vi "Binary MLS.vi"(7 "initialize?":bool=TRUE, 9 "seed":i64=-1 format="%.0x", 10 "polynomial order":i32=31 max=512, 11 "samples":i64=128) -> (0 "error code":i32, 3 "mls sequence":u8[](array[numeric]))   [LabVIEW 2020, in "NI_AALBase.lvlib"]
doc: "Generates a maximum length sequence of ones and zeros using a modulo-2 primitive polynomial of order <B>polynomial order</B>."
uses:
  NI_AALBase.lvlib
panel:
  # "Binary MLS"
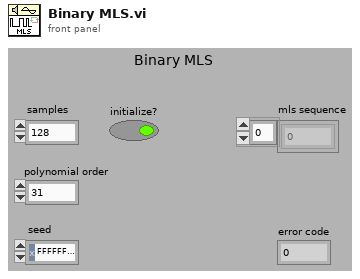
[diagram p1: front panel]
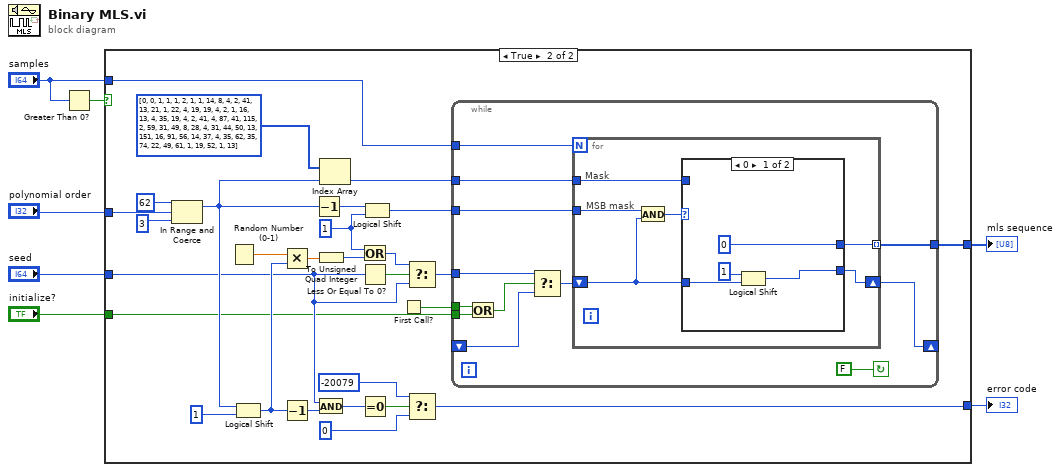
[diagram p0: block diagram]
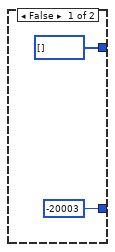
[diagram p2: hidden frame]
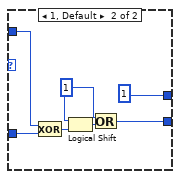
[diagram p3: hidden frame]
diagram:
  n1 = Greater Than 0?(x="samples") -> (x > 0?=w2:bool)
  n2 = case shown="True" w2 {
    tunnel: "polynomial order" -> [_ w35]
    tunnel: "samples" -> [_ w31]
    tunnel: [u8[] [] w28] -> w6
    tunnel: [-20003 ("t") w22] -> w5
    tunnel: "seed" -> [_ w14]
    tunnel: "initialize?" -> [_ w13]
    frame False {
    }
    frame True {
      w16 = u64 1 ("y")
      n3 = In Range and Coerce(upper limit=u16 62, x=w35, lower limit=u16 3) -> (coerced(x)=w25:i32)  [unwired: 1 out]
      n4 = Random Number (0-1)() -> (number: 0 to 1=w18:dbl)
      n5 = Logical Shift(y=w25, x=u64 1 ("y")) -> (x << y=w17:u64)
      n6 = Multiply(x=w18, y=w17) -> (x*y=w20:dbl)
      n7 = Decrement(x=w17) -> (x-1=w26:u64)
      n8 = Decrement(x=w25) -> (x-1=w32:i32)
      n9 = To Unsigned Quad Integer(1:w20) -> (0:w19:u64)
      n10 = And(x=w14, y=w26) -> (x .and. y?=w29:u64)
      n11 = Index Array(array=u64[] [0, 0, 1, 1, 1, 2, 1, 1, 14, 8, 4, 2, 41, 13, 21, 1, 22, 4, 19, 19, 4, 2, 1, 16, 13, 4, 35, 19, 4, 2, 41, 4, 87, 41, 115, 2, 59, 31, 49, 8, 28, 4, 31, 44, 50, 13, 151, 16, 91, 56, 14, 37, 4, 35, 62, 35, 74, 22, 49, 61, 1, 19, 52, 1, 13] ("appended array"), index=w25) -> (element=w34:u64)
      n12 = Or(x=w16, y=w19) -> (x .or. y?=w10:u64)
      n13 = Less Or Equal To 0?(x=w14) -> (x <= 0?=w15:bool)
      n14 = Equal To 0?(x=w29) -> (x = 0?=w24:bool)
      n15 = Logical Shift(y=w32, x=w16) -> (x << y=w33:u64)
      n16 = First Call?() -> (First Call?: T/F=w12:bool)
      n17 = Select(t=w10, s=w15, f=w14) -> (s? t:f=w11:u64)
      n18 = Select(t=-20079, s=w24, f=0) -> (s? t:f=w22:i32)
      n19 = while {
        tunnel: w34 -> [w49]
        tunnel: w33 -> [w48]
        tunnel: w31 -> [w47]
        tunnel: [w46] -> w28
        tunnel: w11 -> [w44]
        shift-right: [w42] -> _
        shift-left: _ -> [w38]
        tunnel: w13 -> [w40]
        tunnel: w12 -> [w41]
        stop <- FALSE continue-if-true
        n20 = Or(x=w41, y=w40) -> (x .or. y?=w39:bool)
        n21 = Select(t=w44, s=w39, f=w38) -> (s? t:f=w43:u64)
        n22 = for {
          N: w47 -> [_]
          shift-right: [w51] -> w42
          shift-left: w43 -> [w50]
          tunnel: w49 -> [w55]
          tunnel: w48 -> [w54]
          tunnel: [w52] -> w46 mode=indexing
          # "MSB mask"
          # "Mask"
          n23 = And(x=w54, y=w50) -> (x .and. y?=w53:u64)
          n24 = case shown="0" w53 {
            tunnel: w50 -> [w59 w65]
            tunnel: w55 -> [_ w66]
            tunnel: [w57 w62] -> w51
            tunnel: [u8 0 ("y") u8 1 ("y")] -> w52
            frame 0 {
              n25 = Logical Shift(y=u32 1, x=w59) -> (x << y=w57:u64)
            }
            frame 1, Default {
              w61 = u64 1 ("y")
              n26 = Exclusive Or(1:w65, 2:w66) -> (0:w64:u64)
              n27 = Logical Shift(y=w61, x=w64) -> (x << y=w63:u64)
              n28 = Or(x=w61, y=w63) -> (x .or. y?=w62:u64)
            }
          }
        }
      }
    }
  }
  "mls sequence" <- w6
  "error code" <- w5
